vi "Simple Crosswalk.vi"() -> ()   [LabVIEW 2023]
uses:
  63daa7d5-0a2c-8f45-ac22-ab1a51a5562e.vi
  091f0f9f-ba83-5e49-bf52-7e477d967a4d.vi
  7815f1a5-79b1-764a-8d89-676041813e43.vi
  04fc8c90-0391-3c46-9268-aa9e1964be30.vi
  <extravilib>/ChannelInstances/One Element Stream-u16/Read With Abort.vi
  <extravilib>/ChannelInstances/One Element Stream-u16/Write With Abort.vi
  <extravilib>/ChannelInstances/One Element Stream-bool/Write With Abort.vi
  <extravilib>/ChannelInstances/One Element Stream-bool/Read With Abort.vi
  <extravilib>/ChannelInstances/One Element Stream-bool/Instantiate.vi
  <extravilib>/ChannelInstances/One Element Stream-u16/Instantiate.vi
  <extravilib>/ChannelInstances/One Element Stream-u16/EndpointRead.vi
  <extravilib>/ChannelInstances/One Element Stream-u16/Endpoint.vi
  <extravilib>/ChannelInstances/One Element Stream-bool/Endpoint.vi
  <extravilib>/ChannelInstances/One Element Stream-bool/EndpointRead.vi
  <extravilib>/ChannelInstances/One Element Stream-bool.lvlib
  <extravilib>/ChannelInstances/One Element Stream-u16.lvlib
panel:
  out "ped":u16(ring)
  out "light":u16(ring)
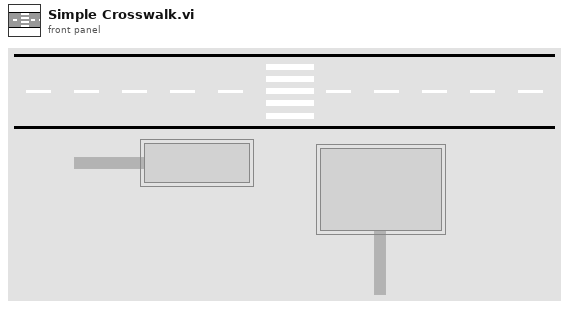
[diagram p1: front panel]
types:
  T1 = typedef "One Element Stream-u16.lvlib/)Channel.ctl" = refnum<queue>
  T2 = typedef "One Element Stream-bool.lvlib/)Channel.ctl" = refnum<queue>
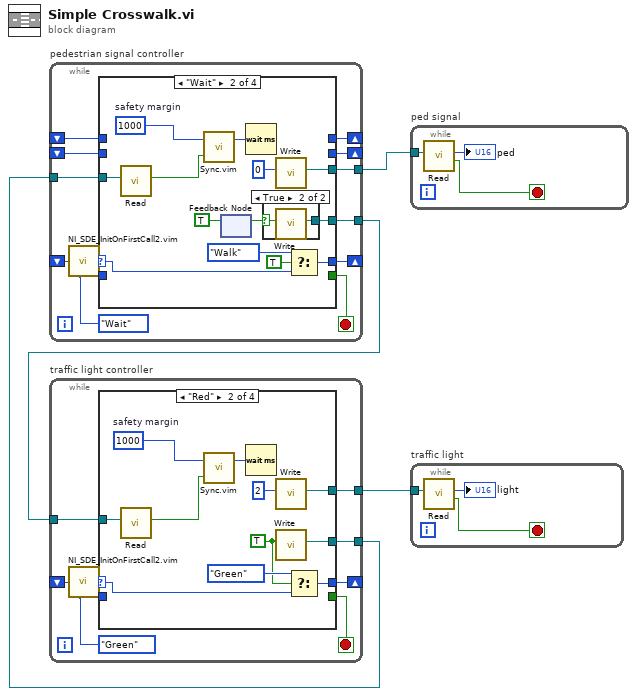
[diagram p0: block diagram]
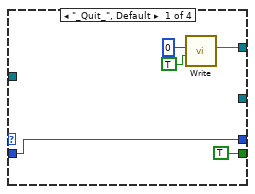
[diagram p2: hidden frame]
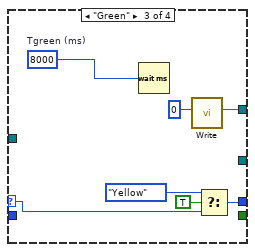
[diagram p3: hidden frame]
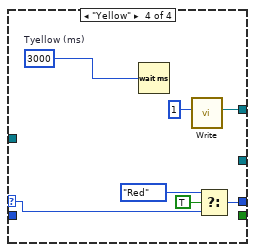
[diagram p4: hidden frame]
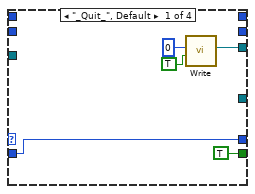
[diagram p5: hidden frame]
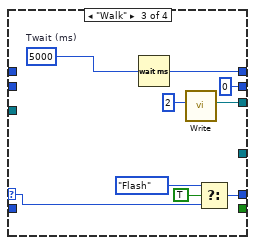
[diagram p7: hidden frame]
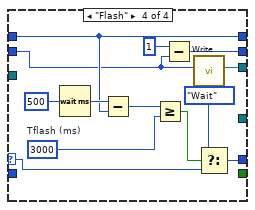
[diagram p8: hidden frame]
diagram:
  n1 = while "pedestrian signal controller" {
    tunnel: w1 -> [w15]
    shift-right: [w14] -> _
    shift-left: _ -> [w13]
    tunnel: [w12] -> w4
    shift-right: [w11] -> _
    shift-left: _ -> [w10]
    tunnel: [w9] -> w2
    shift-right: [w7] -> _
    shift-left: _ -> [w6]
    stop <- w16 stop-if-true
    w8 = enum16{"_Quit_", "Wait", "Walk", "Flash"}."Wait"
    n2 = call "NI_SDE_InitOnFirstCall2.vim"("input"=w6, "master enum"=w8) -> ("output enum"=w5:enum16{"_Quit_", "Wait", "Walk", "Flash"})  [unwired: 1 in]
    n3 = case shown="\"Wait\"" w5 {
      selector: w5 -> [_ w34 w45 w58]
      tunnel: [TRUE _ _ _] -> w16
      tunnel: [w17 w33 w44 w57] -> w7
      tunnel: w15 -> [_ w31 _ _]
      tunnel: [_ _ w40 w51] -> w14
      tunnel: w13 -> [_ _ _ w51]
      tunnel: [w19 w29 w38 w50] -> w12
      tunnel: [_ _ u16 0 w48] -> w11
      tunnel: w10 -> [_ _ _ w47]
      tunnel: [_ w28 _ _] -> w9
      tunnel: w8 -> [w17 _ _ _]
      frame "_Quit_", Default {
        n4 = call <extravilib>:"Write.vi"("last element? (F)"=TRUE, "element"=u16 0) -> ("channel"=w19:T1)  [unwired: 8 in, 1 out]
      }
      frame "Wait" {
        w25 = u32 1000  # safety margin
        n5 = call <extravilib>:"Read.vi"("channel"=w31) -> ("element"=w26:bool)  [unwired: 7 in, 3 out]
        n6 = call "Sync.vim"("a"=w25, "b"=w26) -> ("a'"=w24:u32)  [unwired: 24 in, 1 out]
        n7 = feedback-in #1(TRUE) -> ()
        n8 = feedback #1() -> (w22:bool)  [unwired: 1 in]
        n9 = Wait (ms)(milliseconds to wait=w24) -> ()  [unwired: 1 out]
        n10 = case shown="True" w22 {
          selector: w22 -> [_ w35]
          tunnel: [_ w36] -> w28
          frame False {
          }
          frame True {
            n11 = call <extravilib>:"Write.vi"("element"=w35) -> ("channel"=w36:T2)  [unwired: 9 in, 1 out]
          }
        }
        n12 = call <extravilib>:"Write.vi"("element"=u16 0) -> ("channel"=w29:T1)  [unwired: 9 in, 1 out]
        n13 = Select(t=enum16{"_Quit_", "Wait", "Walk", "Flash"}."Walk", s=TRUE, f=w34) -> (s? t:f=w33:enum16{"_Quit_", "Wait", "Walk", "Flash"})
      }
      frame "Walk" {
        w42 = u32 5000  # Twait (ms)
        n14 = Wait (ms)(milliseconds to wait=w42) -> (millisecond timer value=w40:u32)
        n15 = call <extravilib>:"Write.vi"("element"=u16 2) -> ("channel"=w38:T1)  [unwired: 9 in, 1 out]
        n16 = Select(t=enum16{"_Quit_", "Wait", "Walk", "Flash"}."Flash", s=TRUE, f=w45) -> (s? t:f=w44:enum16{"_Quit_", "Wait", "Walk", "Flash"})
      }
      frame "Flash" {
        w52 = u32 3000  # Tflash (ms)
        n17 = Wait (ms)(milliseconds to wait=u32 500) -> (millisecond timer value=w54:u32)
        n18 = Subtract(x=w54, y=w51) -> (x-y=w53:u32)
        n19 = Greater Or Equal?(x=w53, y=w52) -> (x >= y?=w46:bool)
        n20 = Subtract(x=u16 1, y=w47) -> (x-y=w48:u16)
        n21 = call <extravilib>:"Write.vi"("element"=w47) -> ("channel"=w50:T1)  [unwired: 9 in, 1 out]
        n22 = Select(t=enum16{"_Quit_", "Wait", "Walk", "Flash"}."Wait", s=w46, f=w58) -> (s? t:f=w57:enum16{"_Quit_", "Wait", "Walk", "Flash"})
      }
    }
  }
  n23 = while "traffic light controller" {
    tunnel: w2 -> [w65]
    tunnel: [w64] -> w3
    tunnel: [w63] -> w1
    shift-right: [w60] -> _
    shift-left: _ -> [w61]
    stop <- w66 stop-if-true
    w62 = enum16{"_Quit_", "Red", "Green", "Yellow"}."Green"
    n24 = call "NI_SDE_InitOnFirstCall2.vim"("input"=w61, "master enum"=w62) -> ("output enum"=w59:enum16{"_Quit_", "Red", "Green", "Yellow"})  [unwired: 1 in]
    n25 = case shown="\"Red\"" w59 {
      selector: w59 -> [_ w82 w89 w96]
      tunnel: [TRUE _ _ _] -> w66
      tunnel: [w67 w81 w88 w95] -> w60
      tunnel: w65 -> [_ w79 _ _]
      tunnel: [w69 w77 w83 w93] -> w64
      tunnel: [_ w76 _ _] -> w63
      tunnel: w62 -> [w67 _ _ _]
      frame "_Quit_", Default {
        n26 = call <extravilib>:"Write.vi"("last element? (F)"=TRUE, "element"=u16 0) -> ("channel"=w69:T1)  [unwired: 8 in, 1 out]
      }
      frame "Red" {
        w73 = u32 1000  # safety margin
        w75 = TRUE
        n27 = call <extravilib>:"Read.vi"("channel"=w79) -> ("element"=w74:bool)  [unwired: 7 in, 3 out]
        n28 = call "Sync.vim"("a"=w73, "b"=w74) -> ("a'"=w72:u32)  [unwired: 24 in, 1 out]
        n29 = Wait (ms)(milliseconds to wait=w72) -> ()  [unwired: 1 out]
        n30 = call <extravilib>:"Write.vi"("element"=u16 2) -> ("channel"=w77:T1)  [unwired: 9 in, 1 out]
        n31 = call <extravilib>:"Write.vi"("element"=w75) -> ("channel"=w76:T2)  [unwired: 9 in, 1 out]
        n32 = Select(t=enum16{"_Quit_", "Red", "Green", "Yellow"}."Green", s=w75, f=w82) -> (s? t:f=w81:enum16{"_Quit_", "Red", "Green", "Yellow"})
      }
      frame "Green" {
        w86 = u32 8000  # Tgreen (ms)
        n33 = Wait (ms)(milliseconds to wait=w86) -> ()  [unwired: 1 out]
        n34 = call <extravilib>:"Write.vi"("element"=u16 0) -> ("channel"=w83:T1)  [unwired: 9 in, 1 out]
        n35 = Select(t=enum16{"_Quit_", "Red", "Green", "Yellow"}."Yellow", s=TRUE, f=w89) -> (s? t:f=w88:enum16{"_Quit_", "Red", "Green", "Yellow"})
      }
      frame "Yellow" {
        w90 = u32 3000  # Tyellow (ms)
        n36 = Wait (ms)(milliseconds to wait=w90) -> ()  [unwired: 1 out]
        n37 = call <extravilib>:"Write.vi"("element"=u16 1) -> ("channel"=w93:T1)  [unwired: 9 in, 1 out]
        n38 = Select(t=enum16{"_Quit_", "Red", "Green", "Yellow"}."Red", s=TRUE, f=w96) -> (s? t:f=w95:enum16{"_Quit_", "Red", "Green", "Yellow"})
      }
    }
  }
  n39 = while "ped signal" {
    tunnel: w4 -> [w99]
    stop <- w97 stop-if-true
    n40 = call <extravilib>:"Read.vi"("channel"=w99) -> ("last element?"=w97:bool, "element"=→"ped":u16)  [unwired: 7 in, 2 out]
  }
  n41 = while "traffic light" {
    tunnel: w3 -> [w102]
    stop <- w101 stop-if-true
    n42 = call <extravilib>:"Read.vi"("channel"=w102) -> ("last element?"=w101:bool, "element"=→"light":u16)  [unwired: 7 in, 2 out]
  }
